vi "ConvertTo(boolean).vi"(8 "error in":errorcluster, 9 "Message Payload":variant) -> (0 "error out":errorcluster, 1 "Message Payload boolean":bool)   [LabVIEW 2019]
doc: "Convert variant to boolean\n\nBolder Software LLC"
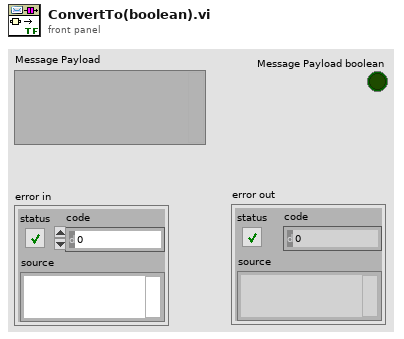
[diagram p1: front panel]
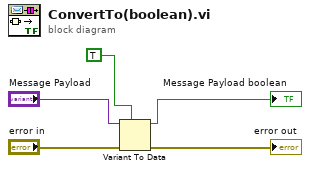
[diagram p0: block diagram]
diagram:
  n1 = Variant To Data(error in="error in", type=TRUE, Variant="Message Payload") -> (data=→"Message Payload boolean":bool, error out=→"error out":errorcluster)
